vi "Get CurrentElementIndex.vi"(8 "error in (no error)":errorcluster, 11 "CircularBuffer":refnum<class "CircularBuffer.lvclass">) -> (0 "error out":errorcluster, 2 "Current Element index":i32=-1, 3 "CircularBuffer out":refnum<class "CircularBuffer.lvclass">)   [LabVIEW 2016, in "CircularBuffer.lvclass"]
doc: "---------------------------------------------------------------\nJKI State Machine Objects™\nhttp://jki.net/state-machine-objects/\nCopyright (C) 2005-2015, JKI <info@jki.net>\nALL RIGHTS RESERVEDJKI State Machine Objects (SMO) 1.0.0.5\nJKI - JKI\nCopyright (c) 2016, JKI"
uses:
  CircularBuffer.lvclass
  CircularBuffer.lvclass/CircularBuffer.ctl
panel:
  # "For instructions on how to use the JKI State Machine Objects, examples and video tutorials, visit:\nhttp://jki.net/state-machine-objects/\n\nJKI State Machine Objects™\nhttp://jki.net/state-machine-objects/\nCopyright (C) 2005-2015, JKI <info@jki.net>\nALL RIGHTS RESERVED"
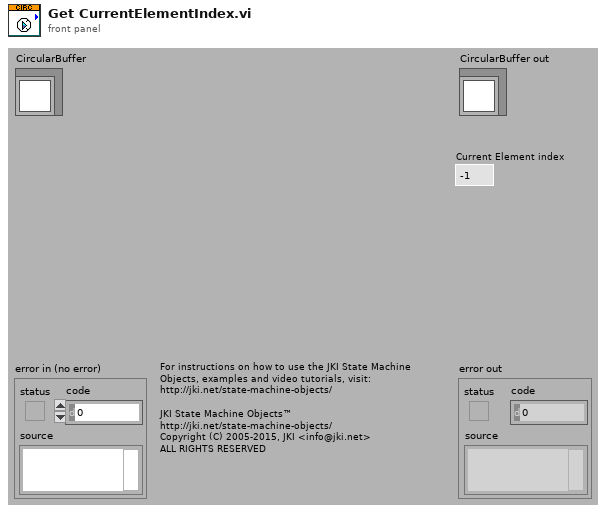
[diagram p1: front panel]
types:
  T1 = typedef "CircularBuffer.lvclass/PrivateData--Ref.ctl" = refnum<data-value>
  T2 = typedef "CircularBuffer.lvclass/PrivateData--Cluster.ctl" = cluster{"Public Events":T3, "Protected Events":T4, "Private Events":T5, "BufferSize":i32, "CurrentElement":i32, "Elements":refnum<data-value>[], "type":refnum<class "type.lvclass">}
  T3 = typedef "CircularBuffer.lvclass/PublicEvents--Cluster.ctl" = cluster{"Buffer Resize Event":refnum<user-event>}
  T4 = typedef "CircularBuffer.lvclass/ProtectedEvents--Cluster.ctl" = cluster{"placeholder":refnum<user-event>}
  T5 = typedef "CircularBuffer.lvclass/PrivateEvents--Cluster.ctl" = cluster{"New Value":refnum<user-event>, "GetElement":refnum<user-event>, "Initialize":refnum<user-event>}
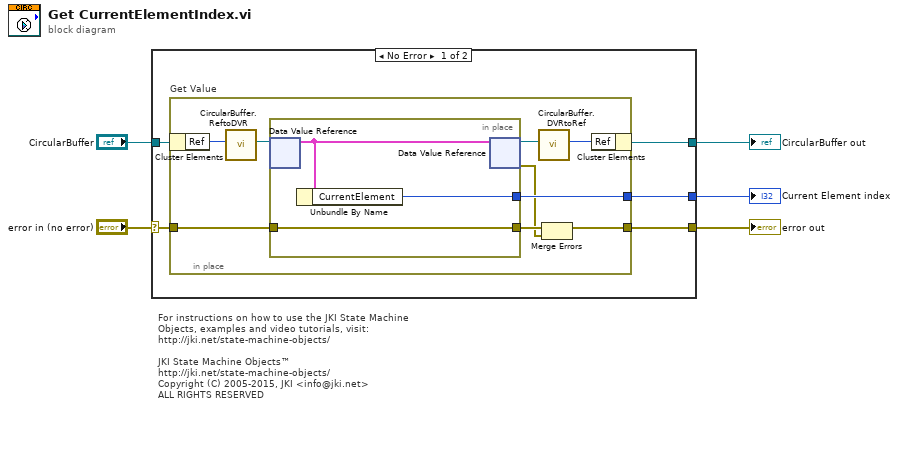
[diagram p0: block diagram]
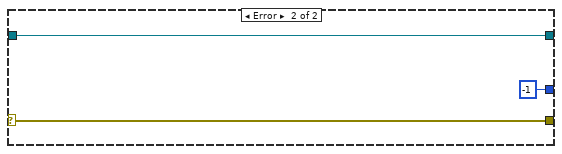
[diagram p2: hidden frame]
diagram:
  # "For instructions on how to use the JKI State Machine Objects, examples and video tutorials, visit:\nhttp://jki.net/state-machine-objects/\n\nJKI State Machine Objects™\nhttp://jki.net/state-machine-objects/\nCopyright (C) 2005-2015, JKI <info@jki.net>\nALL RIGHTS RESERVED"
  n1 = case shown="No Error" "error in (no error)" {
    selector: "error in (no error)" -> [w9 w24]
    tunnel: "CircularBuffer" -> [w10 w25]
    tunnel: [w7 w24] -> w4
    tunnel: [w8 w25] -> w3
    tunnel: [w6 -1] -> w1
    frame No Error {
      n2 = in-place "Get Value" {
        in-place-border: w9 -> [w19]
        in-place-border: [w17] -> w7
        in-place-border: [w16] -> w6
        n3 = in-place-cluster #1(w10) -> ("Ref"=w15:u32)
        n4 = call "CircularBuffer.ReftoDVR.vi"("Ref"=w15) -> ("Ref"=w14:T1)  [unwired: 10 in]
        n5 = in-place {
          in-place-border: w19 -> [w22]
          in-place-border: [w22] -> w18
          in-place-border: [w20] -> w16
          n6 = in-place-dvr #2(w14) -> (w21:T2)  [unwired: 1 out]
          n7 = Unbundle By Name(w21) -> ("CurrentElement"=w20:i32)
          n8 = in-place-dvr #2(w21) -> (w13:T1, w11:errorcluster)
        }
        n9 = call "CircularBuffer.DVRtoRef.vi"("Ref"=w13) -> ("Ref"=w12:u32)  [unwired: 10 in]
        n10 = Merge Errors(w18, w11) -> (w17:errorcluster)
        n11 = in-place-cluster #1("Ref"=w12) -> (w8:refnum<class "CircularBuffer.lvclass">)
      }
    }
    frame Error {
    }
  }
  "error out" <- w4
  "CircularBuffer out" <- w3
  "Current Element index" <- w1
